vi "Configure Is Send Filter.vi"(8 "error in (no error)":errorcluster, 10 "Show Send?":bool, 11 "Debugger In":refnum<class "Debugger.lvclass">) -> (0 "error out":errorcluster, 3 "Debugger Out":refnum<class "Debugger.lvclass">)   [LabVIEW 2020, in "Debugger.lvclass"]
uses:
  Debugger.lvclass
  C:/Users/anton/Documents/GitHub/triarc-debugger/source/Process/Debug Process.lvclass
  Process/Debug Process.lvclass/Debug Process.ctl
  Filter by Is Sender/Filter by Is Send.lvclass
  C:/Users/anton/Documents/GitHub/triarc-debugger/source/Filter by is Action/Filter by Is Action.lvclass
  C:/Users/anton/Documents/GitHub/triarc-debugger/source/Filter/Filter.lvclass
  <vilib>/Utility/error.llb/Clear Errors.vi
  <vilib>/Utility/error.llb/Error Cluster From Error Code.vi
  Debugger.lvclass/Debugger.ctl
  Process/Debug Process.lvclass
  Filter by is Action/Filter by Is Action.lvclass
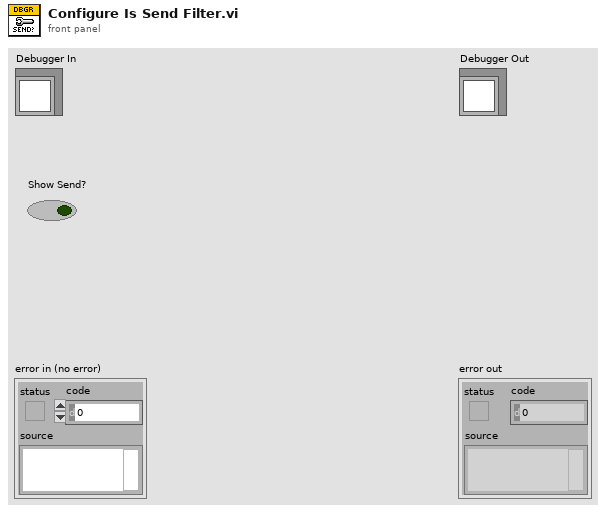
[diagram p1: front panel]
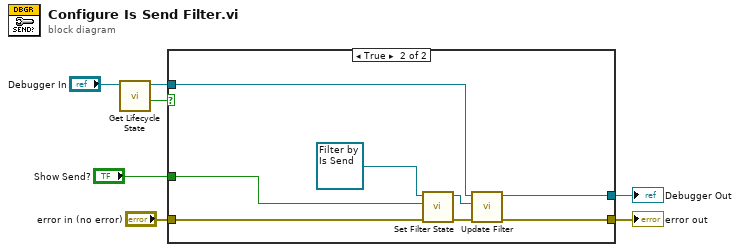
[diagram p0: block diagram]
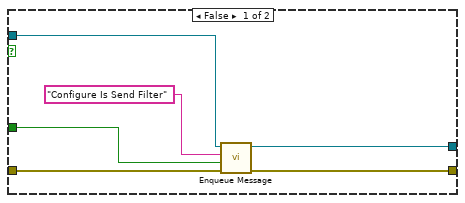
[diagram p2: hidden frame]
diagram:
  n1 = call "Get Lifecycle State.vi"("Process In"="Debugger In") -> ("In Process Loop?"=w2:bool, "Process Out"=w3:refnum<class "Debugger.lvclass">)  [unwired: 7 in, 2 out]
  n2 = case shown="True" w2 {
    tunnel: "error in (no error)" -> [w13 w20]
    tunnel: [w12 w19] -> w6
    tunnel: [w11 w14] -> w4
    tunnel: w3 -> [w9 w21]
    tunnel: "Show Send?" -> [w8 w16]
    frame False {
      n3 = call "Enqueue Message.vi"("error in (no error)"=w13, "Message Data"=w8, "Message"="Configure Is Send Filter", "Process In"=w9) -> ("error out"=w12:errorcluster, "Process Out"=w11:refnum<class "Debugger.lvclass">)  [unwired: 6 in]
    }
    frame True {
      n4 = call "Set Filter State.vi"("error in (no error)"=w20, "Show Action?"=w16, "Filter by Is Action In"=refnum<class "Filter by Is Send.lvclass"> refnum ("Filter by Is Send.lvclass")) -> ("error out"=w17:errorcluster, "Filter by Is Action Out"=w18:refnum<class "Filter by Is Send.lvclass">)  [unwired: 7 in]
      n5 = call "Update Filter.vi"("error in (no error)"=w17, "Filter in"=w18, "Debugger in"=w21) -> ("error out"=w19:errorcluster, "Debugger out"=w14:refnum<class "Debugger.lvclass">)  [unwired: 7 in]
    }
  }
  "error out" <- w6
  "Debugger Out" <- w4
